vi "get broken vi list.vi"() -> (0 "error out":errorcluster, 2 "Broken VI Paths":string[](array[string]), 3 "Broken VI List":string[](array[string]))   [LabVIEW 2020]
doc: "Returns the VIs that are currently broken (would show a broken Run arrow) in the LabVIEW environment G-AI Core is running in, via the Application class's Get Broken VI List method. Takes no input besides the standard error cluster. Run this after creating or editing VIs with the other tools to check whether anything is now broken. Returns two parallel arrays: Broken VI List (each broken VI's bare name, or ClassName.lvclass:VIName.vi if it's a class member) and Broken VI Paths (the same VIs' full absolute file paths) — pass an entry from Broken VI Paths directly as the path argument to get_vi_details or get_project to inspect a specific broken VI further."
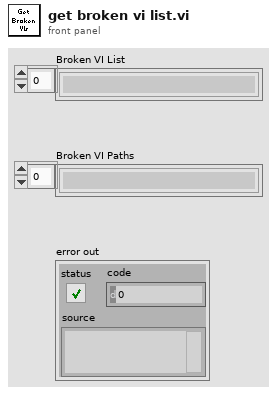
[diagram p1: front panel]
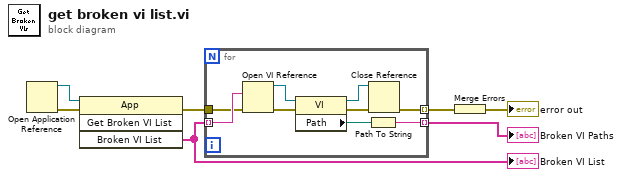
[diagram p0: block diagram]
diagram:
  n1 = Open Application Reference() -> (0:w6:errorcluster, 3:w7:refnum<vi>)  [unwired: 4 in]
  n2 = invoke class="App" method="Get Broken VI List"(reference=w7, error in=w6) -> (error out=w4:errorcluster, "Broken VI List"=w5:string[])  [unwired: 2 in, 2 out]
  "Broken VI List" <- w5
  n3 = for {
    tunnel: w5 -> [w16] mode=indexing
    tunnel: w4 -> [w14]
    tunnel: [w10] -> w2 mode=indexing
    tunnel: [w8] -> w3 mode=indexing
    n4 = Open VI Reference(vi path=w16, error in (no error)=w14) -> (vi reference=w15:refnum<vi>, error out=w13:errorcluster)  [unwired: 4 in]
    n5 = property class="VI"(reference=w15, error in=w13) -> (reference out=w12:refnum<vi>, error out=w11:errorcluster, "Path"=w9:path)
    n6 = Path To String(path=w9) -> (string=w8:string)
    n7 = Close Reference(reference=w12, error in (no error)=w11) -> (error out=w10:errorcluster)
  }
  "Broken VI Paths" <- w3
  n8 = Merge Errors(w2) -> (→"error out":errorcluster)
